vi "Configure Dialog.vi"(8 "error in (no error)":errorcluster, 11 "Configure Channel Msg in":refnum<class "Configure Channel Msg.lvclass">) -> (0 "error out":errorcluster, 2 "Ok?":bool, 3 "Configure Channel Msg out":refnum<class "Configure Channel Msg.lvclass">)   [LabVIEW 2014, in "CS++Scope.lvlib" / "Configure Channel Msg.lvclass"]
uses:
  Configure Channel Msg.lvclass
  Configure Channel Msg.lvclass/Configure Channel Msg.ctl
panel:
  in  "Probe Attenuation":dbl=1.0
  in  "Enabled?":bool
  in  "vertical coupling":i32(ring)=1 caption="Vertical Coupling" items=["AC", "DC", "GND"]
  in  "Vertical Offset":dbl[unit]
  in  "Vertical Range":dbl[unit]
  in  "Channel Name":string="Channel 1"
  in  "OK Button":bool
  in  "Cancel Button":bool
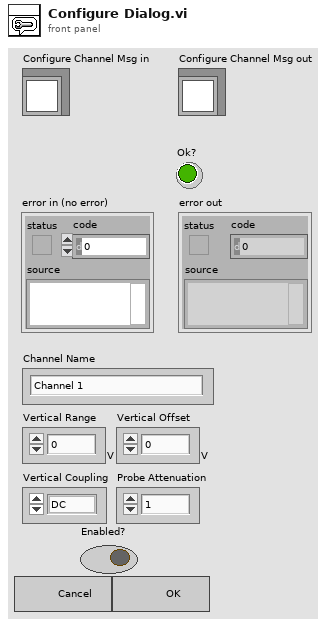
[diagram p1: front panel]
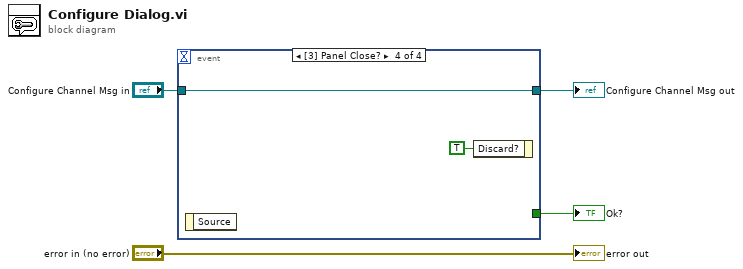
[diagram p0: block diagram]
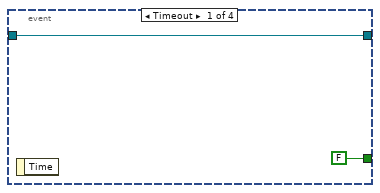
[diagram p2: hidden frame]
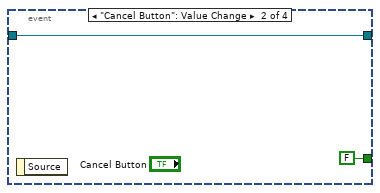
[diagram p3: hidden frame]
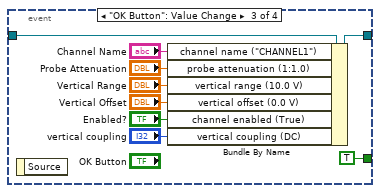
[diagram p4: hidden frame]
diagram:
  n1 = event shown="[3] Panel Close?" {
    selector: _ -> [_ _ _ _]
    dyn-events: _ -> [_ _ _ _]
    timeout: _ -> [_ _ _ _]
    tunnel: [w6 w8 w15 w19] -> w3
    tunnel: "Configure Channel Msg in" -> [w6 w8 w17 w19]
    tunnel: [FALSE FALSE TRUE _] -> w1
    event Timeout {
      n2 = event-data() -> ()  [unwired: 1 in, 1 out]
    }
    event "Cancel Button": Value Change {
      n3 = event-data() -> ()  [unwired: 1 in, 1 out]
    }
    event "OK Button": Value Change {
      n4 = event-data() -> ()  [unwired: 1 in, 1 out]
      n5 = Bundle By Name(cluster=w17, "channel name (\"CHANNEL1\")"="Channel Name", "probe attenuation (1:1.0)"="Probe Attenuation", "vertical range (10.0 V)"="Vertical Range", "vertical offset (0.0 V)"="Vertical Offset", "channel enabled (True)"="Enabled?", "vertical coupling (DC)"="vertical coupling") -> (w15:refnum<class "Configure Channel Msg.lvclass">)
    }
    event Panel Close? {
      n6 = event-data() -> ()  [unwired: 1 in, 1 out]
      n7 = event-data("Discard?"=TRUE) -> ()  [unwired: 1 in, 1 out]
    }
  }
  "Configure Channel Msg out" <- w3
  "Ok?" <- w1
  "error out" <- "error in (no error)"
